vi "class_data.vi"() -> ()   [LabVIEW 2010, in "FPGAWrapperMH120124RAPS_PXI7813R.lvclass"]
uses:
  FPGAWrapperMH120124RAPS_PXI7813R.lvclass
  fpgaVIsAndControls/DDS_board_init_cluster.ctl
  configuration_cluster_raps.ctl
  common_typedefs/channels_cluster.ctl
  fpgaVIsAndControls/ellipsoid_parameters_cluster.ctl
  common_typedefs/gate_parameters_cluster.ctl
  fpgaVIsAndControls/gate_cluster.ctl
  settings_cluster_raps.ctl
panel:
  out "data reader":refnum<k21>
  out "settings writer":refnum<k21>
  in  "# of callers":i32
  out "ready for initialise?":bool=TRUE
  out "allowed to initialise?":bool=TRUE
  out "configuration writer":refnum<k21>
  out "raps writer":refnum<k21>
  out "command writer":refnum<k21>
  # "FSK"
  # "Ramped"
  # "FSK"
  # "Chirp Modus"
  # "Unramped"
  # "BPSK"
  # "Single Tone"
  # "FSK"
  # "Ramped"
  # "FSK"
  # "Chirp Modus"
  # "Unramped"
  # "BPSK"
  # "Single Tone"
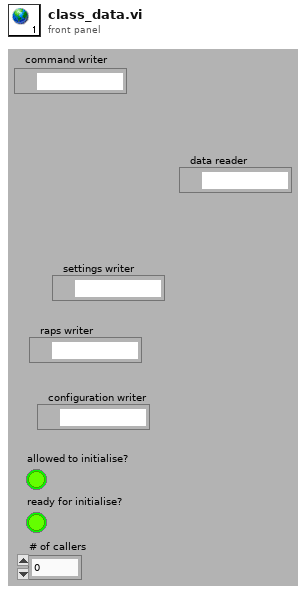
[diagram p1: front panel]
diagram:
